vi "Add Separator Core.vi"(7 "Icon Index (Next)":i32=-1, 8 "error in (no error)":errorcluster, 10 "Image Path":path, 11 "Toolbar Control in":refnum<class "Toolbar Control.lvclass">) -> (0 "error out":errorcluster, 3 "Toolbar Control out":refnum<class "Toolbar Control.lvclass">)   [LabVIEW 2011, in "Toolbar Control.lvclass"]
doc: "This VI is a core which adds a separator provided by path <B>Image Path</B>. This vertical or horizontal separator will be added as an icon that is disabled.\n\n-------------\nDeveloped by Brian Hoover (hooovahh)"
uses:
  Toolbar Control.lvclass
  Toolbar Control.lvclass/Toolbar Control.ctl
  Controls/Button State.ctl
  Controls/Icon Type.ctl
  Controls/Icon Data.ctl
  <vilib>/picture/picture.llb/imagedata.ctl
  <vilib>/Utility/miscctls.llb/LVRectTypeDef.ctl
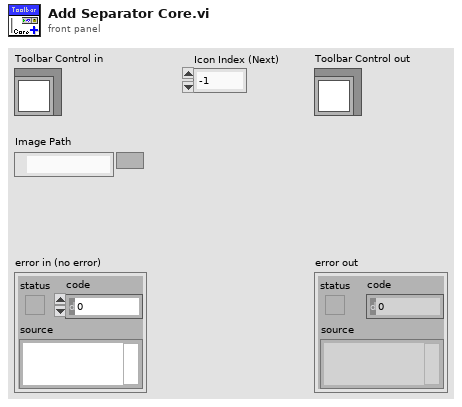
[diagram p1: front panel]
types:
  T1 = typedef "Icon Type.ctl" = enum16{"Normal Icon", "Separator Icon", "More Options"}
  T2 = typedef "Toolbar Control.lvclass/Button State.ctl" = enum8{"Enabled", "Disabled", "Disabled and Grayed Out"}
  T3 = typedef "LVRectTypeDef.ctl" = cluster{"Left":i16, "Top":i16, "Right":i16, "Bottom":i16}
  T4 = typedef "Toolbar Control.lvclass/Icon Data.ctl" = cluster{"Original Image Path":path, "Original Image Data":T5, "Scaled Icon":picture, "Button Name":string, "Button State":T2, "Icon Type":T1}
  T5 = typedef "imagedata.ctl" = cluster{"image type":i32, "image depth":i32, "image":u8[], "mask":u8[], "colors":u32[], "Rectangle":cluster{"left":i16, "top":i16, "right":i16, "bottom":i16}}
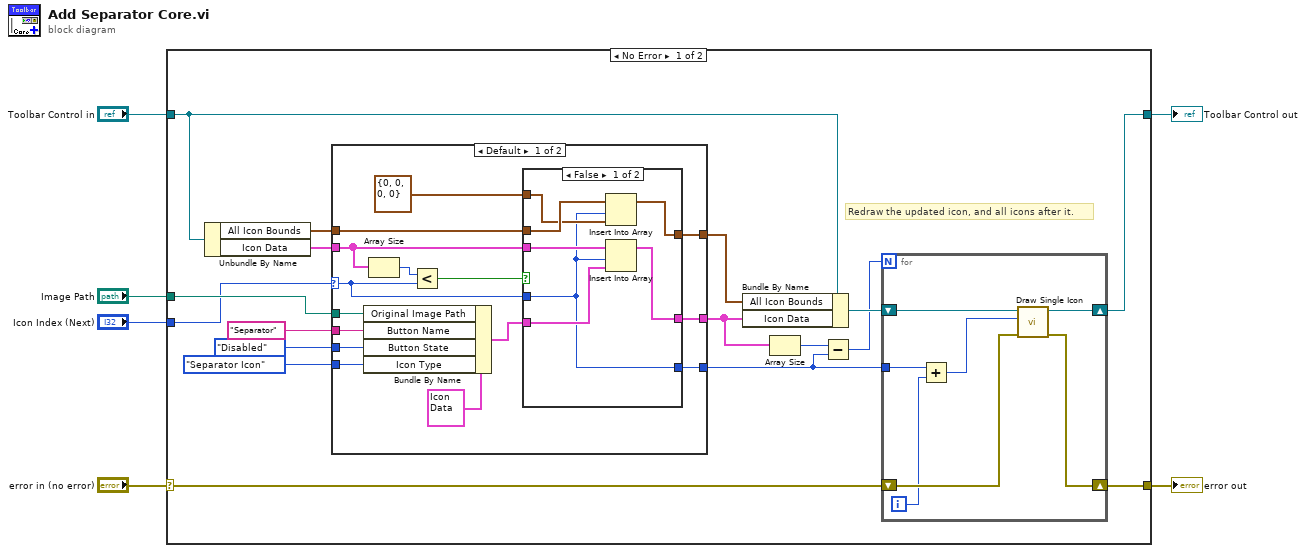
[diagram p0: block diagram]
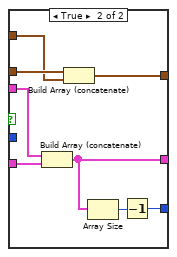
[diagram p2: hidden frame]
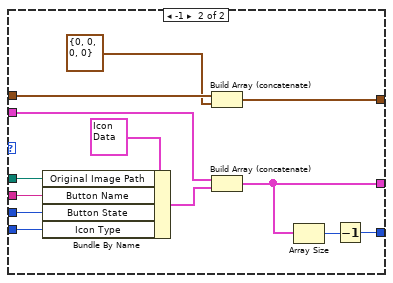
[diagram p3: hidden frame]
diagram:
  n1 = case shown="No Error" "error in (no error)" {
    selector: "error in (no error)" -> [w17 w75]
    tunnel: [w16 w75] -> w5
    tunnel: [w18 w74] -> w3
    tunnel: "Toolbar Control in" -> [w23 w74]
    tunnel: "Image Path" -> [w21 _]
    tunnel: "Icon Index (Next)" -> [w20 _]
    frame No Error {
      # "Redraw the updated icon, and all icons after it."
      n2 = Unbundle By Name(w23) -> ("All Icon Bounds"=w15:T3[], "Icon Data"=w22:T4[])
      n3 = case shown="Default" w20 {
        selector: w20 -> [w37 _]
        tunnel: w21 -> [w45 w72]
        tunnel: "Separator" ("Icon Name") -> [w44 w71]
        tunnel: w22 -> [w42 w70]
        tunnel: [w38 w68] -> w13
        tunnel: [w36 w66] -> w11
        tunnel: w15 -> [w35 w65]
        tunnel: [w34 w63] -> w14
        tunnel: Button_State."Disabled" ("Button State") -> [w32 w62]
        tunnel: Icon_Type."Separator Icon" ("Icon Type") -> [w31 w61]
        frame Default {
          n4 = Bundle By Name(cluster=T4 {"Original Image Path"=path "", "Original Image Data"={"image type"=0, "image depth"=0, "image"=[], "mask"=[], "colors"=[], "Rectangle"={"left"=0, "top"=0, "right"=0, "bottom"=0}}, "Scaled Icon"=bytes[0], "Button Name"="", "Button State"=enum."Enabled", "Icon Type"=enum."Normal Icon"} ("Cluster"), "Original Image Path"=w45, "Button Name"=w44, "Button State"=w32, "Icon Type"=w31) -> (w39:T4)
          n5 = Array Size(array=w42) -> (size(s)=w41:i32)
          n6 = Less?(x=w41, y=w37) -> (x < y?=w40:bool)
          n7 = case shown="False" w40 {
            tunnel: w42 -> [w52 w60]
            tunnel: w39 -> [w51 w59]
            tunnel: [w50 w57] -> w38
            tunnel: w37 -> [w46 _]
            tunnel: [w46 w56] -> w36
            tunnel: w35 -> [w49 w55]
            tunnel: [w48 w54] -> w34
            tunnel: T3 {"Left"=0, "Top"=0, "Right"=0, "Bottom"=0} ("Icon Bounds") -> [w47 w53]
            frame False {
              n8 = Insert Into Array(array=w49, index=w46, new element=w47) -> (w48:T3[])
              n9 = Insert Into Array(array=w52, index=w46, new element=w51) -> (w50:T4[])
            }
            frame True {
              n10 = Build Array (concatenate)(w60, w59) -> (w57:T4[])
              n11 = Build Array (concatenate)(w55, w53) -> (w54:T3[])
              n12 = Array Size(array=w57) -> (size(s)=w58:i32)
              n13 = Decrement(x=w58) -> (x-1=w56:i32)
            }
          }
        }
        frame -1 {
          n14 = Bundle By Name(cluster=T4 {"Original Image Path"=path "", "Original Image Data"={"image type"=0, "image depth"=0, "image"=[], "mask"=[], "colors"=[], "Rectangle"={"left"=0, "top"=0, "right"=0, "bottom"=0}}, "Scaled Icon"=bytes[0], "Button Name"="", "Button State"=enum."Enabled", "Icon Type"=enum."Normal Icon"} ("Cluster"), "Original Image Path"=w72, "Button Name"=w71, "Button State"=w62, "Icon Type"=w61) -> (w69:T4)
          n15 = Build Array (concatenate)(w65, T3 {"Left"=0, "Top"=0, "Right"=0, "Bottom"=0} ("Icon Bounds")) -> (w63:T3[])
          n16 = Build Array (concatenate)(w70, w69) -> (w68:T4[])
          n17 = Array Size(array=w68) -> (size(s)=w67:i32)
          n18 = Decrement(x=w67) -> (x-1=w66:i32)
        }
      }
      n19 = Bundle By Name(cluster=w23, "All Icon Bounds"=w14, "Icon Data"=w13) -> (w19:refnum<class "Toolbar Control.lvclass">)
      n20 = Array Size(array=w13) -> (size(s)=w12:i32)
      n21 = Subtract(x=w12, y=w11) -> (x-y=w10:i32)
      n22 = for {
        N: w10 -> [_]
        tunnel: w11 -> [w26]
        shift-right: [w29] -> w18
        shift-left: w19 -> [w30]
        shift-right: [w27] -> w16
        shift-left: w17 -> [w28]
        i -> [w24]
        n23 = Add(x=w26, y=w24) -> (x+y=w25:i32)
        n24 = call "Draw Single Icon.vi"("error in (no error)"=w28, "Icon Index"=w25, "Toolbar Control in"=w30) -> ("error out"=w27:errorcluster, "Toolbar Control out"=w29:refnum<class "Toolbar Control.lvclass">)  [unwired: 7 in]
      }
    }
    frame Error {
    }
  }
  "error out" <- w5
  "Toolbar Control out" <- w3
